vi "Set_Sweep_Parameter_for_STS.vi"(0 ".NET Reference in":refnum<k24>, 1 "startwave":dbl, 2 "stopwave":dbl, 3 "speed":dbl, 4 "rescalingstep":dbl, 5 "error in (no error)":errorcluster) -> (14 "Reference out":refnum<k24>, 15 "acctualstep":dbl, 19 "error out":errorcluster)   [LabVIEW 2017]
uses:
  C:/Users/Ssantec_Test/Documents/Installment_DLL_Sample_Labview_20211104/DLL/x86/InstrumentDLL.dll
  DLL/x86/InstrumentDLL.dll
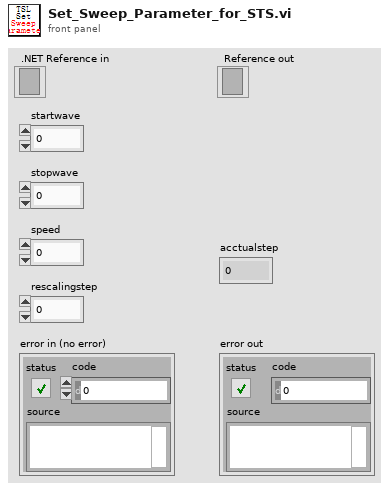
[diagram p1: front panel]
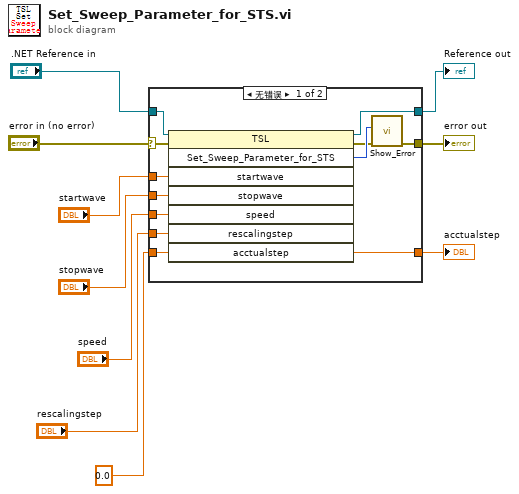
[diagram p0: block diagram]
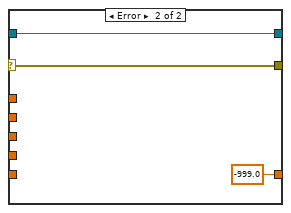
[diagram p2: hidden frame]
diagram:
  n1 = case shown="无错误" "error in (no error)" {
    selector: "error in (no error)" -> [w11 w24]
    tunnel: ".NET Reference in" -> [w22 w25]
    tunnel: [w21 w25] -> w9
    tunnel: [w12 w24] -> w8
    tunnel: [w20 -999.0 ("acctualstep")] -> w7
    tunnel: "startwave" -> [w19 _]
    tunnel: "stopwave" -> [w18 _]
    tunnel: "speed" -> [w17 _]
    tunnel: "rescalingstep" -> [w16 _]
    tunnel: 0.0 ("acctualstep") -> [w15 _]
    frame No Error {
      n2 = invoke on="调用节点" class="TSL" method="Set_Sweep_Parameter_for_STS"(reference=w22, error in=w11, "startwave"=w19, "stopwave"=w18, "speed"=w17, "rescalingstep"=w16, "acctualstep"=w15) -> (reference out=w21:refnum<k24>, error out=w13:errorcluster, "Set_Sweep_Parameter_for_STS"=w14:i32, "acctualstep"=w20:dbl)  [unwired: 1 in, 4 out]
      n3 = call "Show_Error.vi"("error in (no error)"=w13, "Error"=w14) -> ("error out"=w12:errorcluster)  [unwired: 9 in]
    }
    frame Error {
    }
  }
  "Reference out" <- w9
  "error out" <- w8
  "acctualstep" <- w7
